vi "CTRE_CAN_GetFourParam16.vi"(8 "error in (no error)":errorcluster, 11 "ArbID":u32) -> (0 "error out":errorcluster, 2 "4Params":u16[](array[numeric]), 3 "ArbID Out":u32)   [LabVIEW 2016]
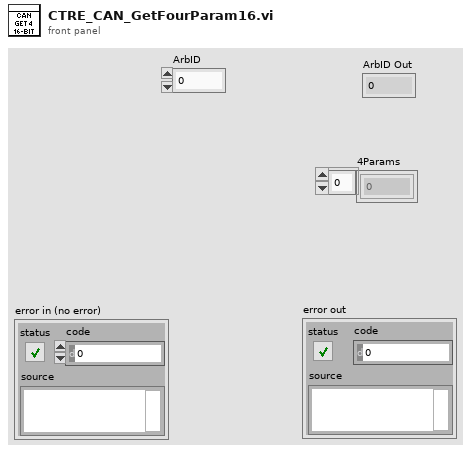
[diagram p1: front panel]
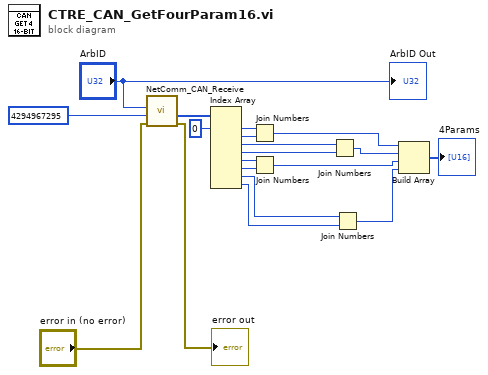
[diagram p0: block diagram]
diagram:
  n1 = call <vilib>:"NetComm_CAN_Receive.vi"("error in (no error)"="error in (no error)", "Message ID Mask"=u32 4294967295, "Message ID"="ArbID") -> ("error out"=→"error out":errorcluster, "Data"=w12:u8[])  [unwired: 5 in, 2 out]
  n2 = Index Array(array=w12, index #1=0 ("index")) -> (element #1=w13:u8, element #2=w14:u8, element #3=w15:u8, element #4=w16:u8, element #5=w17:u8, element #6=w18:u8, element #7=w9:u8, element #8=w8:u8)  [unwired: 7 in]
  n3 = Join Numbers(hi=w13, lo=w14) -> ((hi.lo)=w5:u16)
  n4 = Join Numbers(hi=w17, lo=w18) -> ((hi.lo)=w3:u16)
  n5 = Join Numbers(hi=w15, lo=w16) -> ((hi.lo)=w4:u16)
  n6 = Join Numbers(hi=w9, lo=w8) -> ((hi.lo)=w2:u16)
  n7 = Build Array(w5, w4, w3, w2) -> (→"4Params":u16[])
  "ArbID Out" <- "ArbID"
